vi "Read Binary Config.vi"(4 "Class Name is Included":bool, 6 "byte order (0:big-endian, network order)":T1(ring), 8 "error in (no error)":errorcluster, 10 "Binary":string, 11 "Const_Time in":refnum<class "Const_Time_1D.lvclass">) -> (0 "error out":errorcluster, 2 "Remaining":string, 3 "Const_Time out":refnum<class "Const_Time_1D.lvclass">)   [LabVIEW 2021, in "Const_Time_1D.lvclass"]
uses:
  Const_Time_1D.lvclass
  Const_Time_1D.lvclass/Const_Time_1D.ctl
  Abs_Types/Time 1D/Abs_Time 1D.lvclass
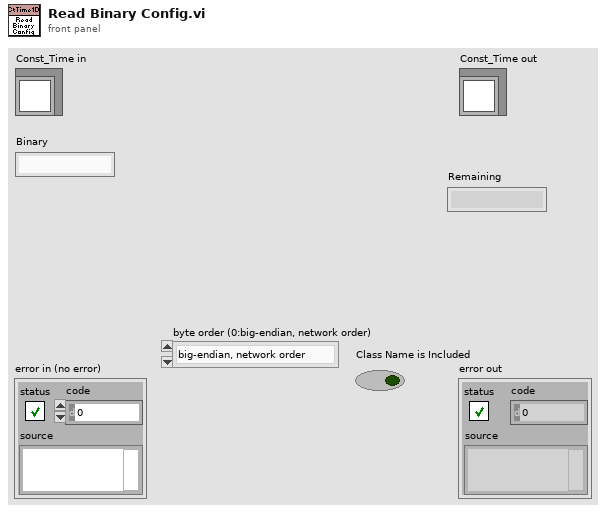
[diagram p1: front panel]
types:
  T1 = enum16{"big-endian, network order", "native, host order", "little-endian"}
  T2 = typedef "Const_Time_1D.lvclass/Type.ctl" = timestamp[]
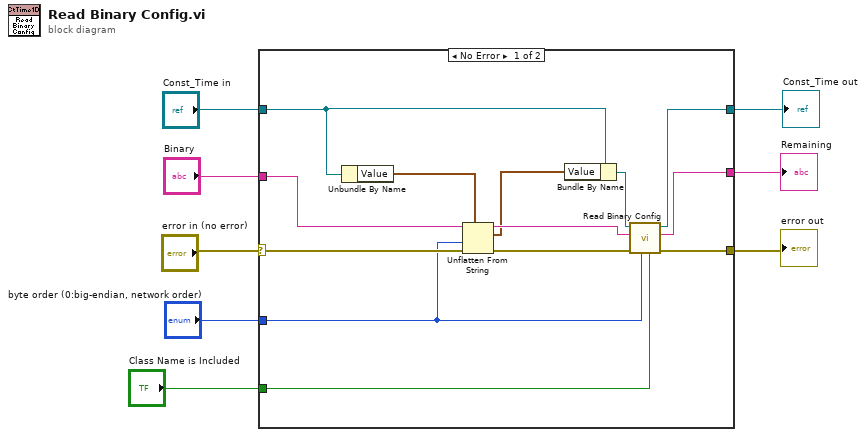
[diagram p0: block diagram]
diagram:
  n1 = case shown="No Error" "error in (no error)" {
    selector: "error in (no error)" -> [w17 w23]
    tunnel: [w21 w23] -> w8
    tunnel: [w20 w24] -> w4
    tunnel: "byte order (0:big-endian, network order)" -> [w11 _]
    tunnel: "Const_Time in" -> [w13 w24]
    tunnel: "Binary" -> [w19 w22]
    tunnel: "Class Name is Included" -> [w10 _]
    tunnel: [w9 w22] -> w1
    frame No Error {
      n2 = Unbundle By Name(w13) -> ("Value"=w12:T2)
      n3 = Unflatten From String(type=w12, binary string=w19, byte order (0:big-endian, network order)=w11, error in (no error)=w17) -> (rest of the binary string=w18:string, value=w14:T2, error out=w16:errorcluster)  [unwired: 1 in]
      n4 = Bundle By Name(cluster=w13, "Value"=w14) -> (w15:refnum<class "Const_Time_1D.lvclass">)
      n5 = call-parent "Read Binary Config.vi"("Class Name is Included"=w10, "byte order (0:big-endian, network order)"=w11, "error in (no error)"=w16, "Binary"=w18, "Abs_Type in"=w15) -> ("error out"=w21:errorcluster, "Remaining"=w9:string, "Abs_Type out"=w20:refnum<class "Const_Time_1D.lvclass">)  [unwired: 4 in]
    }
    frame Error {
    }
  }
  "error out" <- w8
  "Const_Time out" <- w4
  "Remaining" <- w1
